vi "CANOpen_NMR Read config.vi"(8 "error in (no error)":errorcluster, 11 "Section Ref in":T1 format="%.0x") -> (0 "error out":errorcluster, 2 "NMT":T2 {"Node init static SDO state" items=["start remote node"=1, "enter pre-operational"=128]; "Node run state" items=["start remote node"=1, "stop remote node"=2, "enter pre-operational"=128, "reset node"=129, "reset communication"=130]}, 3 "Section Ref out":T1 format="%.0x")   [LabVIEW 2021, in "CANOpen Addon Engine.lvlib"]
uses:
  CANOpen Addon Engine.lvlib
  <vilib>/NI VeriStand/Custom Device API/Custom Device Item Ref.ctl
  CANOpen_NMT Settings.ctl
  Shared/CanOpen_NMT_Config.ctl
  Shared/CanOpen_NMT_Static detect.ctl
  Shared/CANOpen Addon GUID Lookup Global.vi
  <vilib>/NI VeriStand/Custom Device Tools/Custom Device Utility Library/NI VeriStand - Search for Item by GUID.vi
  <vilib>/NI VeriStand/Custom Device API/Get Item Property (Variant).vi
  <vilib>/NI VeriStand/Custom Device API/Custom Device API.lvlib
  Shared/CANOpen Addon Shared.lvlib
  <vilib>/NI VeriStand/Custom Device Tools/Custom Device Utility Library/Custom Device Utility Library.lvlib
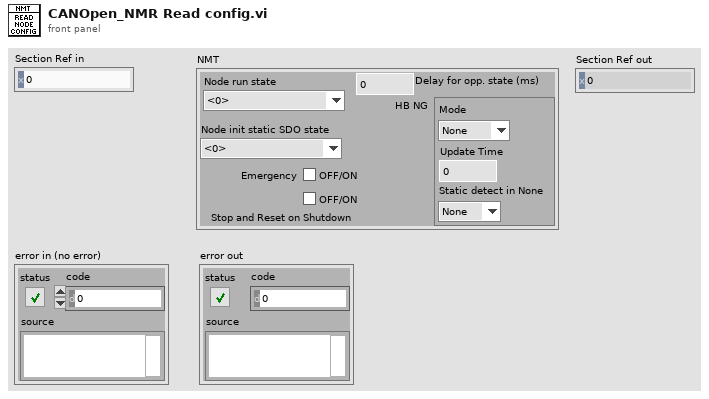
[diagram p1: front panel]
types:
  T1 = typedef "Custom Device API.lvlib/Custom Device Item Ref.ctl" = u64
  T2 = typedef "CANOpen Addon Engine.lvlib/CANOpen_NMT Settings.ctl" = cluster{"Node run state":u16, "Emergency":bool, "HB NG":T3, "Delay for opp. state (ms)":dbl, "Node init static SDO state":u16, "Stop and Reset on Shutdown":bool}
  T3 = typedef "CANOpen Addon Shared.lvlib/CanOpen_NMT_Config.ctl" = cluster{"Mode":T4, "Update Time":u16, "Static detect in None":T4}
  T4 = typedef "CANOpen Addon Shared.lvlib/CanOpen_NMT_Static detect.ctl" = enum16{"None", "HB", "NG"}
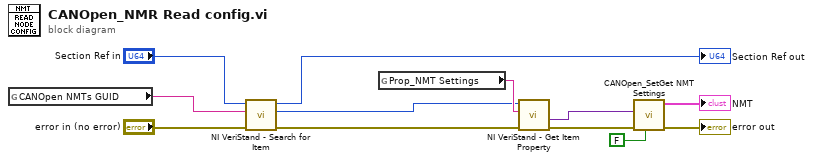
[diagram p0: block diagram]
diagram:
  n1 = global read "CANOpen Addon GUID Lookup Global.vi" "CANOpen NMTs GUID"() -> (w2:string)
  n2 = call-poly <vilib>:"NI VeriStand - Search for Item.vi"("error in"="error in (no error)", "Item GUID"=w2, "Section Ref in"="Section Ref in") -> ("error out"=w5:errorcluster, "Item Ref"=w1:T1, "Section Ref out"=→"Section Ref out":T1)  [unwired: 5 in, 1 out]
  n3 = global read "CANOpen Addon GUID Lookup Global.vi" "Prop_NMT Settings"() -> (w12:string)
  n4 = call-poly <vilib>:"NI VeriStand - Get Item Property.vi"("error in (no error)"=w5, "Property Name"=w12, "Item Ref in"=w1) -> ("error out"=w10:errorcluster, "Value"=w9:variant)  [unwired: 5 in, 2 out]
  n5 = call "CANOpen_SetGet NMT Settings.vi"("Set Parameters"=FALSE, "error in (no error)"=w10, "Parameters"=w9) -> ("error out"=→"error out":errorcluster, "NMT"=→"NMT":T2)  [unwired: 6 in, 1 out]
